vi "FTW-Actor-LocalMessage-CheckShutdown.vi"(0 "FTW-ActorInstance In":refnum<class "FTW-ActorInstance.lvclass">) -> (6 "Shutdown":bool)   [LabVIEW 2013, in "FTW-ActorInstance.lvclass"]
uses:
  FTW-ActorInstance.lvclass
  FTW-ActorInstance.lvclass/FTW-ActorInstance.ctl
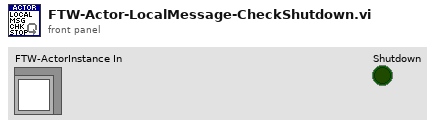
[diagram p1: front panel]
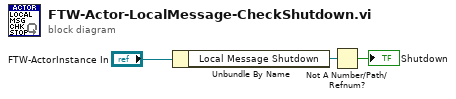
[diagram p0: block diagram]
diagram:
  n1 = Unbundle By Name("FTW-ActorInstance In") -> ("Local Message Shutdown"=w2:refnum<queue>)
  n2 = Not A Number/Path/Refnum?(number/path/refnum=w2) -> (NaN/Path/Refnum?=→"Shutdown":bool)
